vi "Set Dialog Properties.vi"(8 "错误输入（无错误）":cluster{"状态":bool, "代码":i32, "源":string}, 10 "启用对话框属性":bool, 11 "VI引用输入":refnum<vi>) -> (0 "错误输出":cluster{"状态":bool, "代码":i32, "源":string}, 3 "VI引用输出":refnum<vi>)   [LabVIEW 2012]
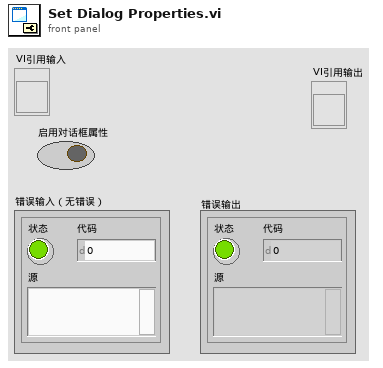
[diagram p1: front panel]
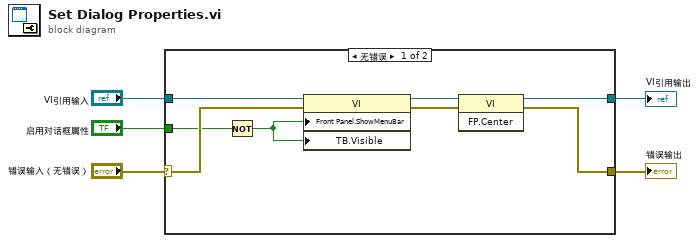
[diagram p0: block diagram]
diagram:
  n1 = case shown="无错误" "错误输入（无错误）" {
    selector: "错误输入（无错误）" -> [w10 w15]
    tunnel: "启用对话框属性" -> [w7 _]
    tunnel: "VI引用输入" -> [w11 w14]
    tunnel: [w9 w14] -> w1
    tunnel: [w8 w15] -> w2
    frame No Error {
      n2 = Not ("非")(x=w7) -> (.not. x?=w6:bool)
      n3 = property on="属性节点" class="VI"(reference=w11, error in=w10, "Front Panel.ShowMenuBar"=w6, "TB.Visible"=w6) -> (reference out=w12:refnum<vi>, error out=w13:errorcluster)
      n4 = invoke on="调用节点" class="VI" method="FP.Center"(reference=w12, error in=w13) -> (reference out=w9:refnum<vi>, error out=w8:errorcluster)  [unwired: 1 in, 1 out]
    }
    frame Error {
    }
  }
  "错误输出" <- w2
  "VI引用输出" <- w1
